vi "configure_sas.vi"(9 "VISA Refnum in":refnum<visa-resource-name>) -> (0 "error out":errorcluster, 3 "VISA Refnum out":refnum<visa-resource-name>)   [LabVIEW 2019]
uses:
  <instrlib>/Agilent E4360/Agilent E4360.lvlib
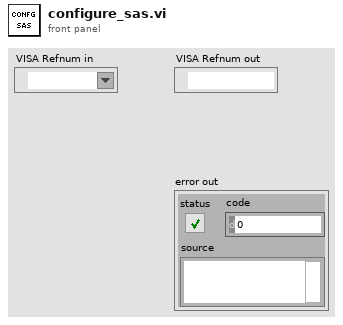
[diagram p1: front panel]
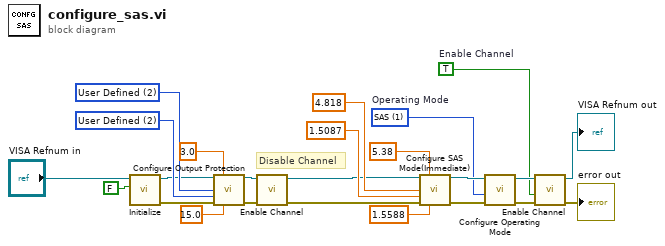
[diagram p0: block diagram]
diagram:
  w9 = 2 items=["MAX", "MIN", "User Defined"] ("Voltage Limit Source (0:MAX)")
  w8 = 2 items=["MAX", "MIN", "User Defined"] ("Current Limit Source (0:MAX)")
  w3 = TRUE  # Enable Channel
  w2 = 1 items=["Fixed", "SAS", "Table"]  # Operating Mode
  # "Disable Channel"
  n1 = call <instrlib>:"Initialize.vi"("ID Query (True)"=FALSE, "VISA resource name"="VISA Refnum in") -> ("error out"=w5:errorcluster, "VISA resource name out"=w4:refnum<visa-resource-name>)  [unwired: 8 in]
  n2 = call <instrlib>:"Configure Output Protection.vi"("VISA resource name"=w4, "Current Limit (0 A)"=3.0, "Current Limit Source (0:MAX)"=w8, "Voltage Limit Source (0:MAX)"=w9, "error in (no error)"=w5, "Voltage Limit (0 V)"=15.0) -> ("VISA resource name out"=w18:refnum<visa-resource-name>, "error out"=w19:errorcluster)  [unwired: 8 in]
  n3 = call <instrlib>:"Enable Channel.vi"("error in (no error)"=w19, "VISA resource name"=w18) -> ("error out"=w11:errorcluster, "VISA resource name out"=w10:refnum<visa-resource-name>)  [unwired: 8 in]
  n4 = call <instrlib>:"Configure SAS Mode(Immediate).vi"("VISA resource name"=w10, "Open Circuit Voltage (0.0 V)"=5.38, "Maximum Voltage Point (0.0 V)"=4.818, "Maximum Current Point (0.0 A)"=1.5087, "error in (no error)"=w11, "Short Circuit Current (0.0 A)"=1.5588) -> ("VISA resource name out"=w16:refnum<visa-resource-name>, "error out"=w17:errorcluster)  [unwired: 8 in]
  n5 = call <instrlib>:"Configure Operating Mode.vi"("error in (no error)"=w17, "Operating Mode (0:Fixed)"=w2, "VISA resource name"=w16) -> ("error out"=w21:errorcluster, "VISA resource name out"=w20:refnum<visa-resource-name>)  [unwired: 7 in]
  n6 = call <instrlib>:"Enable Channel.vi"("error in (no error)"=w21, "Enable Channel (Disable)"=w3, "VISA resource name"=w20) -> ("error out"=→"error out":errorcluster, "VISA resource name out"=→"VISA Refnum out":refnum<visa-resource-name>)  [unwired: 7 in]
